vi "Log Result.vi"(8 "error in (no error)":errorcluster, 9 "Timestamp data points":bool, 10 "Result":refnum<class "Acquired Result.lvclass">, 11 "Logger in":refnum<class "Logger.lvclass">) -> (0 "error out":errorcluster, 3 "Logger out":refnum<class "Logger.lvclass">)   [LabVIEW 2016, in "Logger.lvclass"]
uses:
  Logger.lvclass
  NHMFL_Core/Libraries/Instruments/Results/Acquired Result/Acquired Result.lvclass
  Logger.lvclass/Logger.ctl
  NHMFL_Core/Libraries/File/File Class/File.lvclass/File.ctl
  Read File.lvclass.vi
  Read Last clean-up time stamp.vi
  Read Clean-up period.vi
  NHMFL_Core/Libraries/File/File Class/Write Timestamp data points.vi
  Write File.lvclass.vi
  Write Last clean-up time stamp.vi
  NHMFL_Core/Libraries/File/File Class/File.lvclass
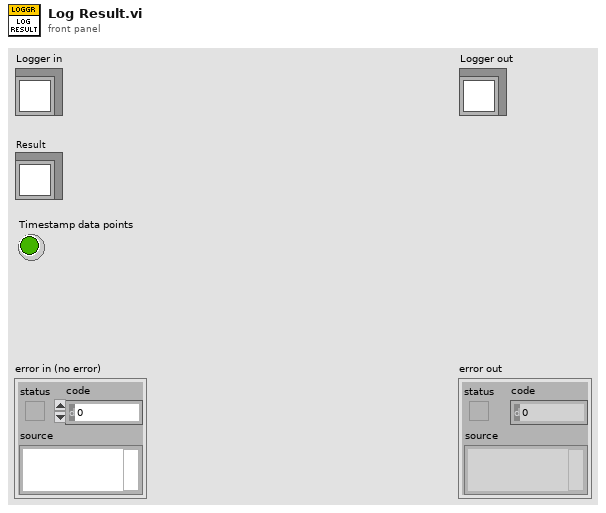
[diagram p1: front panel]
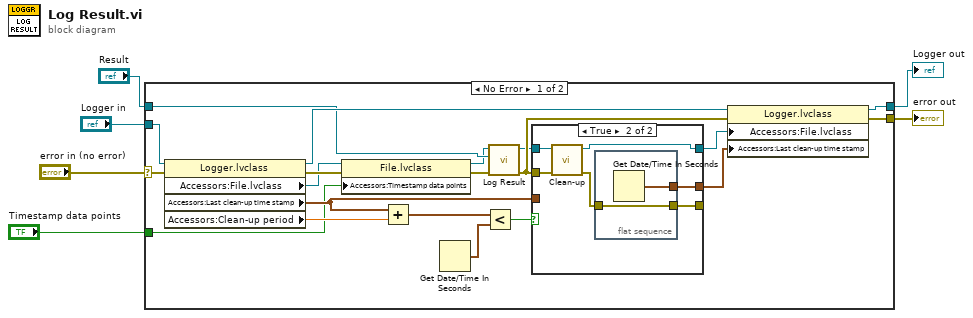
[diagram p0: block diagram]
diagram:
  n1 = case shown="No Error" "error in (no error)" {
    selector: "error in (no error)" -> [w26 w39]
    tunnel: [w24 w39] -> w5
    tunnel: [w22 w38] -> w3
    tunnel: "Logger in" -> [w25 w38]
    tunnel: "Result" -> [w20 _]
    tunnel: "Timestamp data points" -> [w7 _]
    frame No Error {
      n2 = property class="Logger.lvclass"(reference=w25, error in=w26) -> (reference out=w23:refnum<class "Logger.lvclass">, error out=w21:errorcluster, "Accessors:File.lvclass"=w9:refnum<class "File.lvclass">, "Accessors:Last clean-up time stamp"=w12:timestamp, "Accessors:Clean-up period"=w19:dbl)
      n3 = property class="File.lvclass"(reference=w9, error in=w21, "Accessors:Timestamp data points"=w7) -> (reference out=w8:refnum<class "File.lvclass">, error out=w10:errorcluster)
      n4 = Add(x=w12, y=w19) -> (x+y=w17:timestamp)
      n5 = Get Date/Time In Seconds() -> (seconds since 1Jan1904=w18:timestamp)
      n6 = Less?(x=w17, y=w18) -> (x < y?=w16:bool)
      n7 = call-dynamic "Log Result.vi"("error in (no error)"=w10, "Result"=w20, "File in"=w8) -> ("error out"=w15:errorcluster, "File out"=w14:refnum<class "File.lvclass">)  [unwired: 7 in]
      n8 = case shown="True" w16 {
        tunnel: w15 -> [w29 w35]
        tunnel: w14 -> [w28 w34]
        tunnel: [w29 w30] -> _
        tunnel: [w28 w33] -> w13
        tunnel: w12 -> [w27 _]
        tunnel: [w27 w32] -> w11
        frame False {
        }
        frame True {
          n9 = call-dynamic "Clean-up.vi"("error in (no error)"=w35, "File in"=w34) -> ("error out"=w31:errorcluster, "File out"=w33:refnum<class "File.lvclass">)  [unwired: 8 in]
          n10 = flat-sequence {
            tunnel: [w37] -> w32
            tunnel: w31 -> [w36]
            tunnel: [w36] -> w30
            frame #0 {
              n11 = Get Date/Time In Seconds() -> (seconds since 1Jan1904=w37:timestamp)
            }
          }
        }
      }
      n12 = property class="Logger.lvclass"(reference=w23, error in=w15, "Accessors:File.lvclass"=w13, "Accessors:Last clean-up time stamp"=w11) -> (reference out=w22:refnum<class "Logger.lvclass">, error out=w24:errorcluster)
    }
    frame Error {
    }
  }
  "error out" <- w5
  "Logger out" <- w3
